vi "Selftest Device Core.vi"(8 "error in (no error)":errorcluster, 11 "KIT-QVA in":refnum<class "KIT-QVA.lvclass">) -> (0 "error out":errorcluster, 1 "Self-Test Result Message":string, 2 "Self-Test Result Code":i32, 3 "KIT-QVA out":refnum<class "KIT-QVA.lvclass">)   [LabVIEW 2016, in "KIT-QVA.lvlib" / "KIT-QVA.lvclass"]
doc: "Perform selftest of device."
uses:
  KIT-QVA.lvclass
  KIT-QVA.lvclass/KIT-QVA.ctl
  CSPP_Core/Actors/CS++DeviceActor/CS++DeviceActor.lvclass
  instr.lib/KIT-QV/KIT QV.lvlib
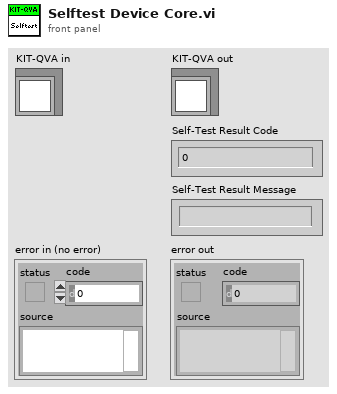
[diagram p1: front panel]
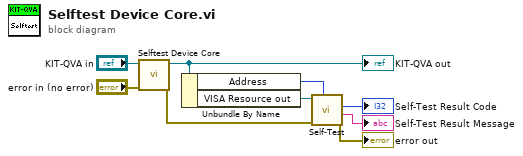
[diagram p0: block diagram]
diagram:
  n1 = call-parent "Selftest Device Core.vi"("error in (no error)"="error in (no error)", "CS++DeviceActor in"="KIT-QVA in") -> ("error out"=w4:errorcluster, "CS++DeviceActor out"=w7:refnum<class "KIT-QVA.lvclass">)  [unwired: 6 in, 2 out]
  "KIT-QVA out" <- w7
  n2 = Unbundle By Name(w7) -> ("Address"=w5:u16, "VISA Resource out"=w6:refnum<visa-resource-name>)
  n3 = call "Self-Test.vi"("Address"=w5, "Error In"=w4, "VISA Resource in"=w6) -> ("Error Out"=→"error out":errorcluster, "Self-Test Result Message"=→"Self-Test Result Message":string, "Self-Test Result Code"=→"Self-Test Result Code":i32)  [unwired: 5 in, 1 out]
